vi "ObtainQueue.vi"(8 "ErrorArray":errorcluster[](array[cluster])) -> (0 "ErrorArray":errorcluster[](array[cluster]), 2 "QueueRef":refnum<queue>)   [LabVIEW 2014, in "Queue.lvlib"]
uses:
  Queue.lvlib
  clMessage.ctl
  <userlib>/NIST/NISTErrorLib/NISTErrorLib.lvlib
panel:
  # "This obtaind a queue and\nenqueues the \"Initialize\"\nMessage"
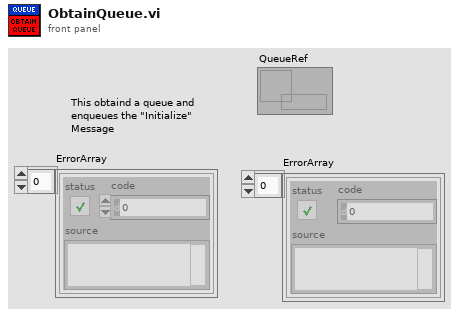
[diagram p1: front panel]
types:
  T1 = typedef "Queue.lvlib/clMessage.ctl" = cluster{"Message":string, "Message Data":variant}
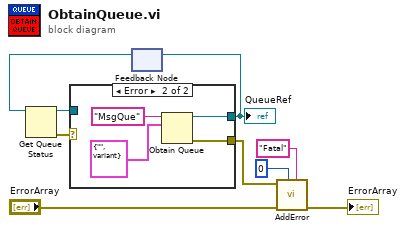
[diagram p0: block diagram]
diagram:
  n1 = feedback #1() -> (w5:refnum<queue>)  [unwired: 1 in]
  n2 = Get Queue Status(queue=w5) -> (queue out=w3:refnum<queue>, error out=w4:errorcluster)  [unwired: 2 in, 6 out]
  n3 = case shown="Error" w4 {
    tunnel: [_ w12] -> w2
    tunnel: [w10 w11] -> w1
    tunnel: w3 -> [w10 _]
    frame No Error {
    }
    frame Error {
      n4 = Obtain Queue(name (unnamed)="MsgQue", element data type=T1 {"Message"="", "Message Data"=variant} ("clMessage")) -> (queue out=w11:refnum<queue>, error out=w12:errorcluster)  [unwired: 3 in, 1 out]
    }
  }
  "QueueRef" <- w1
  n5 = feedback-in #1(w1) -> ()
  n6 = call <userlib>:"AddError.vi"("Severity"="Fatal", "Priority"=u8 0, "ErrorArray"="ErrorArray", "error in (no error)"=w2) -> ("ErrorArray"=→"ErrorArray":errorcluster[])  [unwired: 6 in, 1 out]
